vi "Strip Spaces.vi"(10 "input string":string) -> (2 "result string":string)   [LabVIEW 2013]
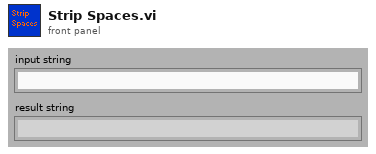
[diagram p1: front panel]
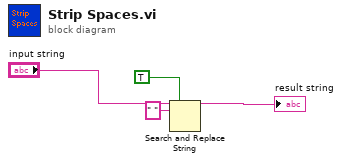
[diagram p0: block diagram]
diagram:
  n1 = Search and Replace String(replace all?=TRUE ("replace all? (F)"), input string="input string", search string=" ") -> (result string=→"result string":string)  [unwired: 1 in, 7 out]
